vi "zlock_release.vi"(8 "error in (no error)":errorcluster, 10 "key":string, 11 "ZLock in":T1) -> (0 "error out":errorcluster, 2 "key out":string, 3 "ZLock out":T1)   [LabVIEW 2010]
uses:
  <userlib>/BIAS2/subvis/zlock/zlock.ctl
  <vilib>/addons/zeromq/zmq_context.lvclass
panel:
  out "reply":string
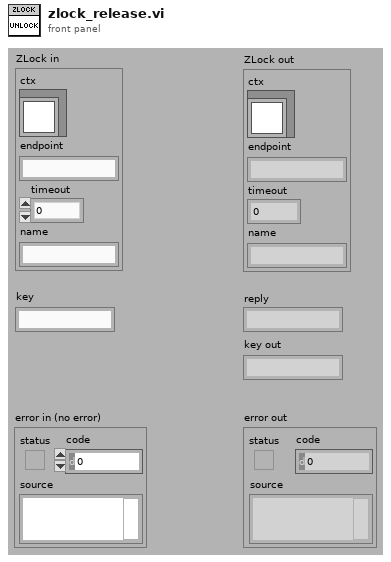
[diagram p1: front panel]
types:
  T1 = typedef "zlock.ctl" = cluster{"ctx":refnum<class "zmq_context.lvclass">, "endpoint":string, "timeout":u32, "name":string}
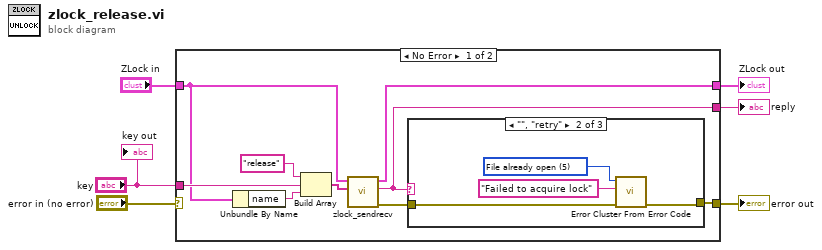
[diagram p0: block diagram]
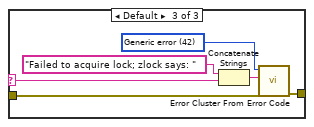
[diagram p3: hidden frame]
diagram:
  n1 = case shown="No Error" "error in (no error)" {
    selector: "error in (no error)" -> [_ w28]
    tunnel: [w13 w28] -> w5
    tunnel: [w8 w27] -> w3
    tunnel: "ZLock in" -> [w7 w27]
    tunnel: "key" -> [w12 _]
    tunnel: [w9 _] -> w1
    frame No Error {
      n2 = Unbundle By Name(w7) -> ("name"=w14:string)
      n3 = Build Array("release" ("data"), w12, w14) -> (w11:string[])
      n4 = call <userlib>:"zlock_sendrecv.vi"("parts"=w11, "socket in"=w7) -> ("error out"=w10:errorcluster, "reply"=w9:string, "socket out"=w8:T1)  [unwired: 7 in]
      n5 = case shown="\"\", \"retry\"" w9 {
        selector: w9 -> [_ _ w22]
        tunnel: [w16 w20 w26] -> w13
        tunnel: w10 -> [w16 w17 w21]
        frame "ok" {
        }
        frame "", "retry" {
          w19 = 5 items=["No error", "Argument error", "Memory is full", "Out of zone", "End of file", "File already open", "Generic file I/O error", "File not found", "File permission error", "Disk is full", "Duplicate path", "Too many files open", "System feature not enabled", "Resource file not found", "Cannot add resource", "Resource not found", "Image not found", "Image memory error", "Pen does not exist", "Config type invalid", "Config token not found", "Config parse error", "Config memory error", "Bad external code format", "Bad external code offset", "External code not present", "Null window", "Destroy window error", "Null menu", "Print aborted", "Bad print record", "Print driver error", "Windows error during printing", "Memory error during printing", "Print dialog error", "Generic print error", "Invalid device refnum", "Device not found", "Device parameter error", "Device unit error", "Cannot open device", "Device call aborted", "Generic error", "Cancelled by user", "Object ID too low", "Object ID too high", "Object not in heap", "Unknown heap", "Unknown object (invalid DefProc)", "Unknown object (DefProc not in table)", "Message out of range", "Invalid (null) method", "Unknown message", "Manager call not supported", "Bad address", "Network operation in progress", "Network operation timed out", "Connection is busy", "Network attribute not supported", "Network error", "Address in use", "System out of memory", "Connection aborted", "Connection refused", "Not connected", "Already connected", "Connection closed", "Initialization error (interapplication manager)", "Bad occurrence", "Wait on unbound occurrence handler", "Occurrence queue overflow", "Datalog type conflict", "Unused", "Unrecognized type (interapplication manager)", "Memory corrupt", "Failed to make temporary DLL", "Old CIN version", "Drag socket not found", "Failed to load drop-object", "Failed to register OLE object", "Failed to release OLE object", "Format specifier type mismatch", "Unknown format specifier", "Too few format specifiers", "Too many format specifiers", "Scan failed", "Newer CIN version", "Error converting to variant", "Runtime menu error", "Password tampered", "Variant attribute not found", "Incompatible variant data type", "Event data is not available", "Event Store is not present", "Occurrence is not found", "Event Queue is not created", "Event info is not available", "Refnum passed is NULL", "Error retrieving Class GUID", "Error retrieving CoClass GUID", "Error retrieving TypeLib GUID.", "Bad built application magic bytes.", "Specific driver is different from the specific driver associated with the Logical Name.", "There is no session opened to the class driver.", "Max Error", "MAX - Error with config objects", "MAX - Error loading configuration", "MAX - Group not supported"]
          n6 = call <vilib>:"Error Cluster From Error Code.vi"("error in (no error)"=w17, "error message (\"\")"="Failed to acquire lock" ("error message (\"\")"), "error code (0)"=w19) -> ("error out"=w20:errorcluster)  [unwired: 6 in]
        }
        frame Default {
          w25 = 42 items=["No error", "Argument error", "Memory is full", "Out of zone", "End of file", "File already open", "Generic file I/O error", "File not found", "File permission error", "Disk is full", "Duplicate path", "Too many files open", "System feature not enabled", "Resource file not found", "Cannot add resource", "Resource not found", "Image not found", "Image memory error", "Pen does not exist", "Config type invalid", "Config token not found", "Config parse error", "Config memory error", "Bad external code format", "Bad external code offset", "External code not present", "Null window", "Destroy window error", "Null menu", "Print aborted", "Bad print record", "Print driver error", "Windows error during printing", "Memory error during printing", "Print dialog error", "Generic print error", "Invalid device refnum", "Device not found", "Device parameter error", "Device unit error", "Cannot open device", "Device call aborted", "Generic error", "Cancelled by user", "Object ID too low", "Object ID too high", "Object not in heap", "Unknown heap", "Unknown object (invalid DefProc)", "Unknown object (DefProc not in table)", "Message out of range", "Invalid (null) method", "Unknown message", "Manager call not supported", "Bad address", "Network operation in progress", "Network operation timed out", "Connection is busy", "Network attribute not supported", "Network error", "Address in use", "System out of memory", "Connection aborted", "Connection refused", "Not connected", "Already connected", "Connection closed", "Initialization error (interapplication manager)", "Bad occurrence", "Wait on unbound occurrence handler", "Occurrence queue overflow", "Datalog type conflict", "Unused", "Unrecognized type (interapplication manager)", "Memory corrupt", "Failed to make temporary DLL", "Old CIN version", "Drag socket not found", "Failed to load drop-object", "Failed to register OLE object", "Failed to release OLE object", "Format specifier type mismatch", "Unknown format specifier", "Too few format specifiers", "Too many format specifiers", "Scan failed", "Newer CIN version", "Error converting to variant", "Runtime menu error", "Password tampered", "Variant attribute not found", "Incompatible variant data type", "Event data is not available", "Event Store is not present", "Occurrence is not found", "Event Queue is not created", "Event info is not available", "Refnum passed is NULL", "Error retrieving Class GUID", "Error retrieving CoClass GUID", "Error retrieving TypeLib GUID.", "Bad built application magic bytes.", "Specific driver is different from the specific driver associated with the Logical Name.", "There is no session opened to the class driver.", "Max Error", "MAX - Error with config objects", "MAX - Error loading configuration", "MAX - Group not supported"]
          n7 = Concatenate Strings("Failed to acquire lock; zlock says: " ("error message (\"\")"), w22) -> (w23:string)
          n8 = call <vilib>:"Error Cluster From Error Code.vi"("error in (no error)"=w21, "error message (\"\")"=w23, "error code (0)"=w25) -> ("error out"=w26:errorcluster)  [unwired: 6 in]
        }
      }
    }
    frame Error {
    }
  }
  "error out" <- w5
  "ZLock out" <- w3
  "reply" <- w1
  "key out" <- "key"
